vi "WSVCAP SHL Host LL RFFE Build and Parse Read Message.vi"(0 "Write Data In":u8[][](array[numeric]) format="%.0x", 1 "Message In":string, 7 "Status In":u8[](array[numeric]), 11 "error in":errorcluster) -> (3 "Message Out":string, 4 "Write Data Out":u8[][](array[numeric]) format="%.0x", 8 "Status":u8[](array[numeric]), 15 "error out":errorcluster)   [LabVIEW 2012]
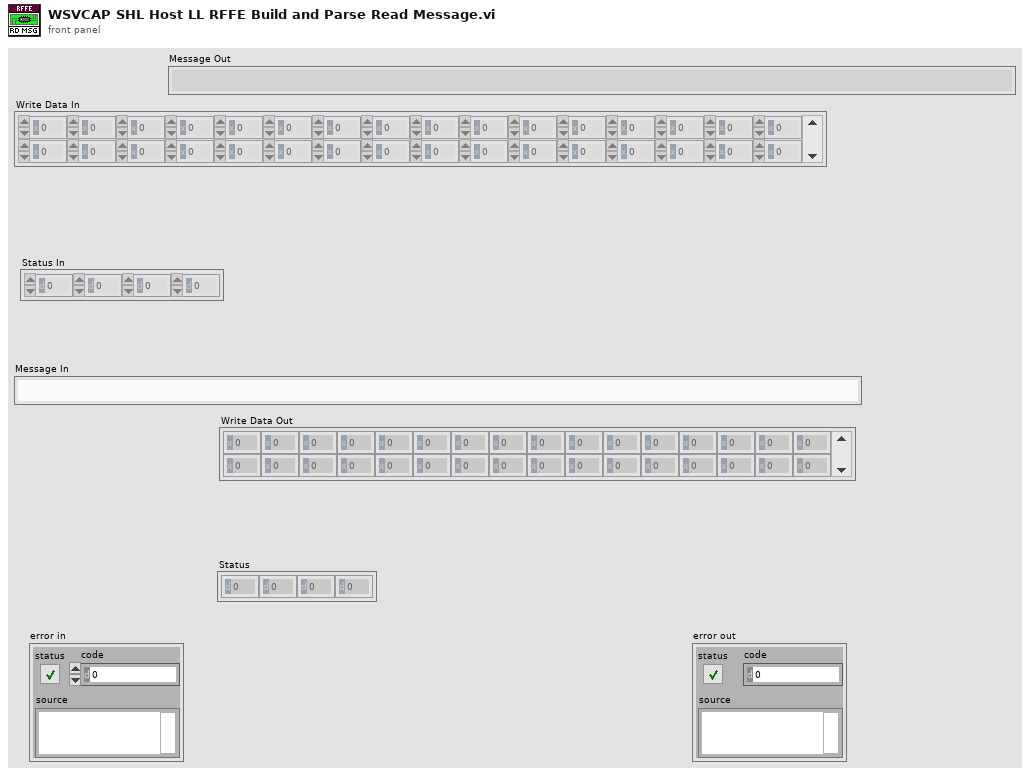
[diagram p1: front panel]
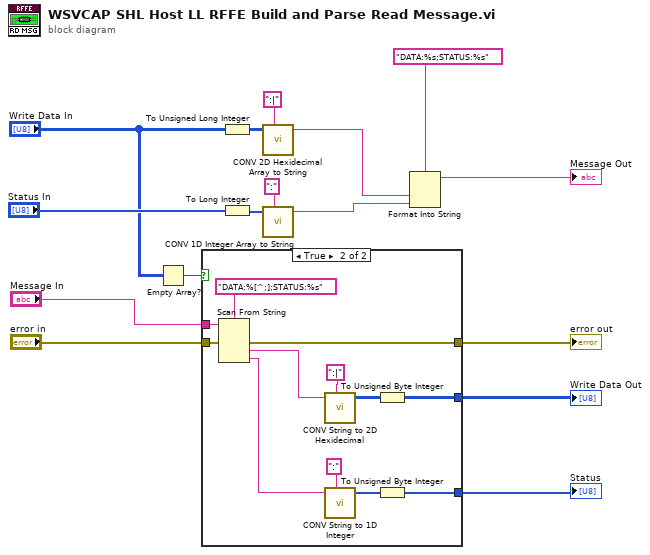
[diagram p0: block diagram]
diagram:
  n1 = Empty Array?(array="Write Data In") -> (empty?=w1:bool)
  n2 = case shown="True" w1 {
    tunnel: [_ w28] -> w12
    tunnel: "error in" -> [w17 w24]
    tunnel: [w17 w23] -> w10
    tunnel: [_ w19] -> w6
    tunnel: "Message In" -> [_ w18]
    frame False {
    }
    frame True {
      n3 = Scan From String(format string="DATA:%[^;];STATUS:%s", input string=w18, error in=w24) -> (error out=w23:errorcluster, output 1=w26:string, output 2=w22:string)  [unwired: 3 in, 2 out]
      n4 = call "CONV String to 2D Hexidecimal.vi"("String"=w26, "Delimiters (,;)"=":|") -> ("2-D Hexidecimal"=w29:u32[][])  [unwired: 7 in]
      n5 = call "CONV String to 1D Integer.vi"("String"=w22, "Delimiter (,)"=":" ("Delimiters (,;)")) -> ("1-D Integer"=w20:i32[])  [unwired: 7 in]
      n6 = To Unsigned Byte Integer(number=w29) -> (unsigned 8bit integer=w28:u8[][])
      n7 = To Unsigned Byte Integer(number=w20) -> (unsigned 8bit integer=w19:u8[])
    }
  }
  "Write Data Out" <- w12
  "error out" <- w10
  "Status" <- w6
  n8 = To Unsigned Long Integer(number="Write Data In") -> (unsigned 32bit integer=w16:u32[][])
  n9 = To Long Integer(number="Status In") -> (32bit integer=w8:i32[])
  n10 = call "CONV 2D Hexidecimal Array to String.vi"("2-D Hexidecimal"=w16, "Delimiters (,;)"=":|") -> ("String"=w15:string)  [unwired: 7 in]
  n11 = call "CONV 1D Integer Array to String.vi"("1-D Integer"=w8, "Delimiter (,)"=":" ("Delimiters (,;)")) -> ("String"=w7:string)  [unwired: 7 in]
  n12 = Format Into String(format string="DATA:%s;STATUS:%s", w15, w7) -> (resulting string=→"Message Out":string)  [unwired: 2 in, 1 out]
